vi "cal.vi"(8 "array":dbl[](array[numeric]), 9 "Laser Wavelength":dbl, 10 "Wave Number":dbl[](array[numeric]), 11 "Pixel":dbl[](array[numeric])) -> (1 "array 2":dbl[](array[numeric]), 2 "Result":dbl[](array[numeric]))   [LabVIEW 2014]
uses:
  <vilib>/express/express arith-compare/Formula/XNode/ExpressFormulaBlockNode.xnode
  <vilib>/Analysis/NI_AALPro.lvlib
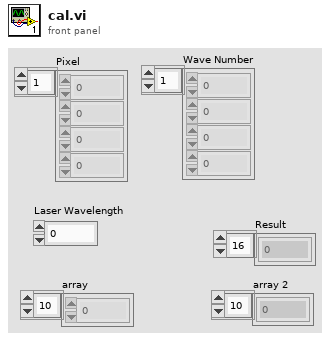
[diagram p1: front panel]
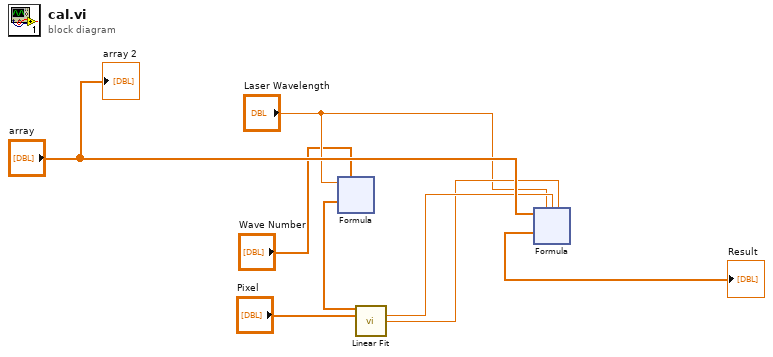
[diagram p0: block diagram]
diagram:
  n1 = xnode ("Formula")("X1"="Laser Wavelength", "X2"="Wave Number") -> ("Result"=w1:dbl[])  [unwired: 1 in, 1 out]
  n2 = call <vilib>:"Linear Fit.vi"("Y"=w1, "X"="Pixel") -> ("slope"=w5:dbl, "intercept"=w4:dbl)  [unwired: 9 in, 3 out]
  n3 = xnode "Formula"("X1"="array", "X2"="Laser Wavelength", "X3"=w5, "X4"=w4) -> ("Result"=→"Result":dbl[])  [unwired: 1 in, 1 out]
  "array 2" <- "array"
